vi "test_csm_lumikki_instron_startRamp.vi"   [LabVIEW 2009]
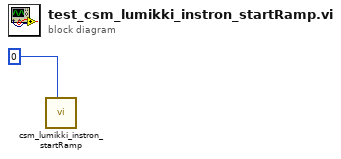
[diagram p0: block diagram]
diagram:
  n1 = call "csm_lumikki_instron_startRamp.vi"("ChannelInt"=0) -> ()  [unwired: 11 in]
